vi "Get CEID Data.vi"(8 "error in (no error)":errorcluster, 11 "CEID":u32) -> (0 "error out":errorcluster, 2 "OK?":bool, 3 "S6F16":T1)   [LabVIEW 2020, in "SECS Scenarios.lvlib" / "08-Host Requsts Event Report.lvclass"]
uses:
  08-Host Requsts Event Report.lvclass
  SECS Communication/S6 Message Class/S6F16.ctl
  SECS Communication/SECS-II Class/Format Code.ctl
  SECS Communication/SECS Data Class/Get RPTID Data.vi
  SECS Communication/SECS Data Class/Get SVID Data.vi
  SECS Communication/SECS Data Class/Get ECID Data.vi
  SECS Communication/SECS Data Class/Get ALID Data.vi
  SECS Communication/SECS Data Class/SECS Data Class.lvclass
  SECS Communication/SECS-II Class/SECS-II Class.lvclass
  SECS Communication/S6 Message Class/S6 Message Class.lvclass
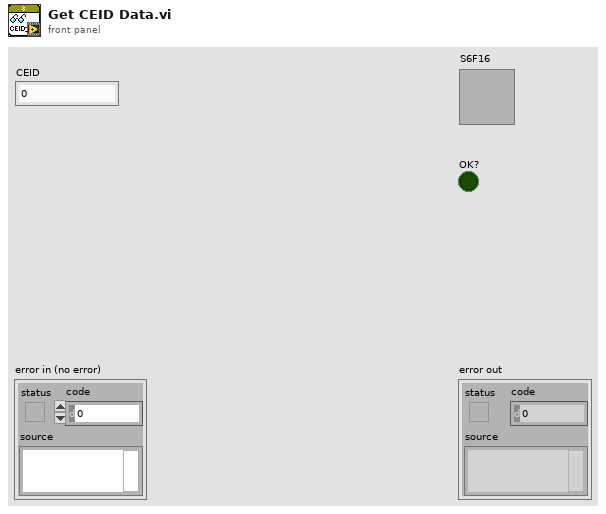
[diagram p1: front panel]
types:
  T1 = typedef "SECS Communication.lvlib/S6 Message Class.lvclass/S6F16.ctl" = cluster{"DATAID":u32, "CEID":u32, "Report Data":cluster{"RPTID":u32, "Value":cluster{"Format Code":T2, "Value":variant}[]}[]}
  T2 = typedef "SECS Communication.lvlib/SECS-II Class.lvclass/Format Code.ctl" = enum16{"L", "A", "B", "Boolean", "J", "I1", "I2", "I4", "I8", "U1", "U2", "U4", "U8", "F4", "F8", "Char"}
  T3 = typedef "SECS Communication.lvlib/SECS Data Class.lvclass/CEID Data.ctl" = cluster{"Enable":bool, "CEID":u32, "Name":string, "Description":string, "RPTID":u32[], "Dynamic":bool}
  T4 = typedef "SECS Communication.lvlib/SECS Data Class.lvclass/RPTID Data.ctl" = cluster{"RPTID":u32, "Report Information":string[], "Dynamic":bool}
  T5 = typedef "SECS Communication.lvlib/SECS Data Class.lvclass/SVID Data.ctl" = cluster{"SVID":u32, "Name":string, "Description":string, "Format Code":T2, "Unit":string, "Source":string, "Data":variant}
  T6 = typedef "SECS Communication.lvlib/SECS Data Class.lvclass/ECID Data.ctl" = cluster{"ECID":u32, "Name":string, "Description":string, "Format Code":T2, "Unit":string, "Max":dbl, "Min":dbl, "Default":string, "Source":string, "Data":variant}
  T7 = typedef "SECS Communication.lvlib/SECS Data Class.lvclass/ALID Data.ctl" = cluster{"Enable":bool, "ALID":u32, "Name":string, "Description":string, "Source":string, "Status":enum16{"Null", "Normal", "Abnormal", "Warning"}}
  T8 = cluster{"RPTID":u32, cluster{"Format Code":T2, "Variant":variant}[]}
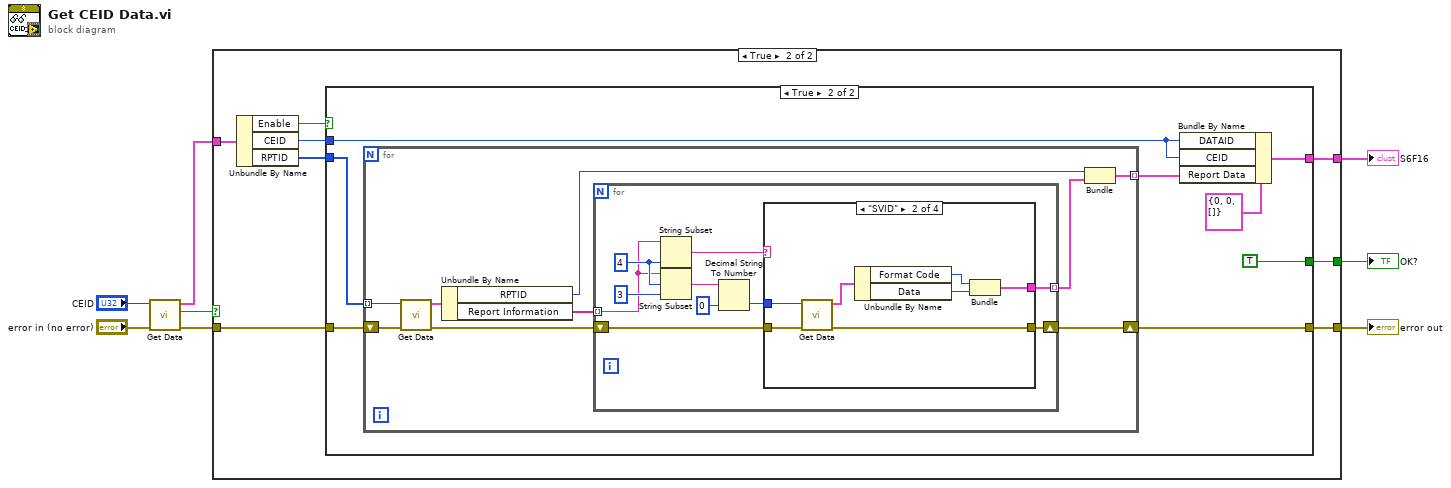
[diagram p0: block diagram]
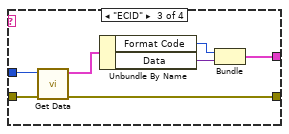
[diagram p5: hidden frame]
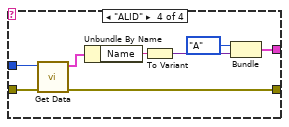
[diagram p6: hidden frame]
diagram:
  n1 = call-poly "Get Data.vi"("error in"="error in (no error)", "CEID"="CEID") -> ("error out"=w8:errorcluster, "Find?"=w7:bool, "CEID Data"=w6:T3)  [unwired: 7 in]
  n2 = case shown="True" w7 {
    tunnel: w8 -> [w9 w16]
    tunnel: w6 -> [_ w17]
    tunnel: [w9 w13] -> w2
    tunnel: [_ w12] -> w1
    tunnel: [_ w11] -> w3
    frame False {
    }
    frame True {
      n3 = Unbundle By Name(w17) -> ("Enable"=w10:bool, "CEID"=w14:u32, "RPTID"=w15:u32[])
      n4 = case shown="True" w10 {
        tunnel: w16 -> [w18 w26]
        tunnel: w15 -> [_ w25]
        tunnel: w14 -> [_ w24]
        tunnel: [w18 w23] -> w13
        tunnel: [_ TRUE] -> w12
        tunnel: [_ w21] -> w11
        frame False {
        }
        frame True {
          n5 = for {
            shift-right: [w31] -> w23
            shift-left: w26 -> [w35]
            tunnel: w25 -> [w30] mode=indexing
            tunnel: [w27] -> w20 mode=indexing
            n6 = call-poly "Get Data.vi"("error in"=w35, "RPTID"=w30) -> ("error out"=w33:errorcluster, "RPTID Data"=w34:T4)  [unwired: 7 in, 1 out]
            n7 = Unbundle By Name(w34) -> ("RPTID"=w28:u32, "Report Information"=w32:string[])
            n8 = for {
              shift-right: [w37] -> w31
              shift-left: w33 -> [w39]
              tunnel: w32 -> [w36] mode=indexing
              tunnel: [w38] -> w29 mode=indexing
              w45 = 4 ("length (rest)")
              n9 = String Subset(string=w36, length (rest)=w45) -> (substring=w41:string)  [unwired: 1 in]
              n10 = String Subset(string=w36, offset (0)=w45, length (rest)=3 ("length (rest)")) -> (substring=w43:string)
              n11 = Decimal String To Number(string=w43, default (0L)=u32 0 ("default (0 I32)")) -> (number=w40:u32)  [unwired: 1 in, 1 out]
              n12 = case shown="\"SVID\"" w41 {
                tunnel: w40 -> [_ w52 w59 w64]
                tunnel: w39 -> [w46 w53 w60 w65]
                tunnel: [_ w48 w55 w68] -> w38
                tunnel: [w46 w47 w54 w63] -> w37
                frame Default {
                }
                frame "SVID" {
                  n13 = call-poly "Get Data.vi"("error in"=w53, "SVID"=w52) -> ("error out"=w47:errorcluster, "SVID Data"=w51:T5)  [unwired: 7 in, 1 out]
                  n14 = Unbundle By Name(w51) -> ("Format Code"=w49:T2, "Data"=w50:variant)
                  n15 = Bundle("Format Code"=w49, "Data"=w50) -> (w48:cluster{"Format Code":T2, "Data":variant})  [unwired: 1 in]
                }
                frame "ECID" {
                  n16 = call-poly "Get Data.vi"("error in"=w60, "ECID"=w59) -> ("error out"=w54:errorcluster, "ECID Data"=w58:T6)  [unwired: 7 in, 1 out]
                  n17 = Unbundle By Name(w58) -> ("Format Code"=w56:T2, "Data"=w57:variant)
                  n18 = Bundle("Format Code"=w56, "Data"=w57) -> (w55:cluster{"Format Code":T2, "Data":variant})  [unwired: 1 in]
                }
                frame "ALID" {
                  n19 = call-poly "Get Data.vi"("error in"=w65, "ALID"=w64) -> ("error out"=w63:errorcluster, "ALID Data"=w62:T7)  [unwired: 7 in, 1 out]
                  n20 = Unbundle By Name(w62) -> ("Name"=w61:string)
                  n21 = To Variant(anything=w61) -> (Variant=w66:variant)
                  n22 = Bundle("Format Code"=Format_Code."A", "Variant"=w66) -> (w68:cluster{"Format Code":T2, "Variant":variant})  [unwired: 1 in]
                }
              }
            }
            n23 = Bundle("RPTID"=w28, w29) -> (w27:T8)  [unwired: 1 in]
          }
          n24 = Bundle By Name(cluster=T1 {"DATAID"=0, "CEID"=0, "Report Data"=[]} ("S6F16"), "DATAID"=w24, "CEID"=w24, "Report Data"=w20) -> (w21:T1)
        }
      }
    }
  }
  "error out" <- w2
  "S6F16" <- w3
  "OK?" <- w1
